vi "IP-1.vi"(0 "array":bool[](array[boolean])) -> (1 "Right":bool[](array[boolean]), 2 "Left":bool[](array[boolean]))   [LabVIEW 2013]
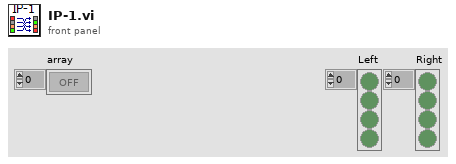
[diagram p1: front panel]
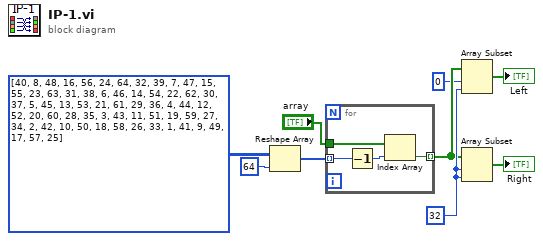
[diagram p0: block diagram]
diagram:
  w6 = 32 ("length")
  n1 = Reshape Array(u8[][] [[40, 8, 48, 16, 56, 24, 64, 32], [39, 7, 47, 15, 55, 23, 63, 31], [38, 6, 46, 14, 54, 22, 62, 30], [37, 5, 45, 13, 53, 21, 61, 29], [36, 4, 44, 12, 52, 20, 60, 28], [35, 3, 43, 11, 51, 19, 59, 27], [34, 2, 42, 10, 50, 18, 58, 26], [33, 1, 41, 9, 49, 17, 57, 25]], 64 ("dimension size")) -> (w8:u8[])
  n2 = for {
    tunnel: "array" -> [w12]
    tunnel: w8 -> [w13] mode=indexing
    tunnel: [w10] -> w3 mode=indexing
    n3 = Decrement(x=w13) -> (x-1=w11:u8)
    n4 = Index Array(array=w12, index=w11) -> (element=w10:bool)
  }
  n5 = Array Subset(array=w3, index=0, length=w6) -> (→"Left":bool[])
  n6 = Array Subset(array=w3, index=w6, length=w6) -> (→"Right":bool[])
